vi "_API_BINANCE_GET_USDT_FUTURES_QueryOrder.vi"(0 "BinanceAPI in":refnum<class "BinanceAPI_.lvclass">, 5 "QueryOrder":T1={"symbol"="NaN", "orderId"=nan, "origClientOrderId"="NaN", "recvWindow"=5000}, 11 "error in (no error)":errorcluster) -> (4 "BinanceAPI out":refnum<class "BinanceAPI_.lvclass">, 14 "Body":string, 15 "error out":errorcluster)   [LabVIEW 2022 SP3, in "BinanceAPI_.lvclass"]
doc: "https://binance-docs.github.io/apidocs/futures/en/#new-order-trade"
uses:
  BinanceAPI_.lvclass
  BinanceAPI_.lvclass/BinanceAPI_.ctl
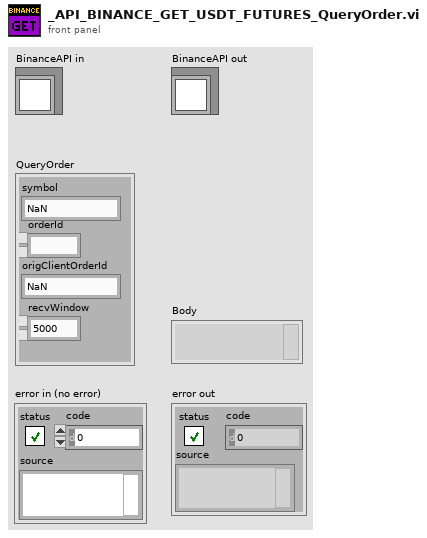
[diagram p1: front panel]
types:
  T1 = cluster{"symbol":string, "orderId":ext, "origClientOrderId":string, "recvWindow":i32}
  T2 = enum16{"SPOT", "USDT_FUTURES", "COIN_FUTURES", "VANILLA"}
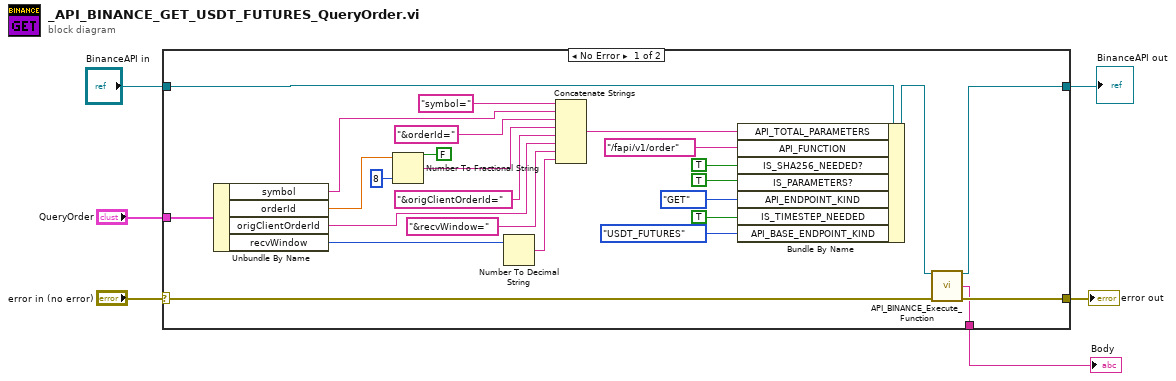
[diagram p0: block diagram]
diagram:
  n1 = case shown="No Error" "error in (no error)" {
    selector: "error in (no error)" -> [w25 w34]
    tunnel: [w21 w34] -> w5
    tunnel: [w22 w33] -> w1
    tunnel: "BinanceAPI in" -> [w26 w33]
    tunnel: "QueryOrder" -> [w29 _]
    tunnel: [w7 _] -> w3
    frame No Error {
      n2 = Unbundle By Name(w29) -> ("symbol"=w18:string, "orderId"=w15:ext, "origClientOrderId"=w13:string, "recvWindow"=w9:i32)
      n3 = Number To Fractional String(use system decimal point (T)=FALSE, number=w15, precision (6)=i16 8) -> (F-format string=w16:string)  [unwired: 1 in]
      n4 = Number To Decimal String(number=w9) -> (decimal integer string=w8:string)  [unwired: 1 in]
      n5 = Concatenate Strings("symbol=" ("Symbol"), w18, "&orderId=" ("Symbol"), w16, "&origClientOrderId=" ("Symbol"), w13, "&recvWindow=" ("Symbol"), w8) -> (w28:string)
      n6 = Bundle By Name(cluster=w26, "API_TOTAL_PARAMETERS"=w28, "API_FUNCTION"="/fapi/v1/order", "IS_SHA256_NEEDED?"=TRUE, "IS_PARAMETERS?"=TRUE, "API_ENDPOINT_KIND"=enum16{"POST", "DELETE", "GET", "PUT"}."GET", "IS_TIMESTEP_NEEDED"=TRUE ("IS_PARAMETERS?"), "API_BASE_ENDPOINT_KIND"=T2."USDT_FUTURES") -> (w23:refnum<class "BinanceAPI_.lvclass">)
      n7 = call "API_BINANCE_Execute_Function.vi"("BinanceAPI in"=w23, "error in (no error)"=w25) -> ("BinanceAPI out"=w22:refnum<class "BinanceAPI_.lvclass">, "Body"=w7:string, "error out"=w21:errorcluster)  [unwired: 9 in, 2 out]
    }
    frame Error {
    }
  }
  "error out" <- w5
  "Body" <- w3
  "BinanceAPI out" <- w1
